vi "Create Summary File.vi"(7 "FP":T1, 8 "error in":errorcluster, 11 "Report":T2) -> (0 "error out":errorcluster, 1 "Vac?":bool, 2 "Pass/Fail":bool, 3 "resulting string":string)   [LabVIEW 2018]
uses:
  Results.ctl
  Vacuum Test.ctl
  Vacuum Output.ctl
  Main Refs.ctl
  Hardware/Tecan/Pump Config.ctl
  Vacuum Specs.ctl
  Cartridges.ctl
  Cartridge Status.ctl
  Commands.ctl
  Lib/Time/Wells.ctl
  Lib/Time/Bottles.ctl
  Process State.ctl
  Main Globals.vi
panel:
  # "Tecan Pump"
  # "Vacuum"
  # "General"
  # "Protocol"
  # "Zaber"
  # "NFC Reader 1"
  # "NFC  Reader 2"
  # "NFC Reader 3"
  # "NFC Reader 4"
  # "System"
  # "Cartridge Utitlies"
  # "Wells"
  # "times"
  # "from"
  # "State Machine"
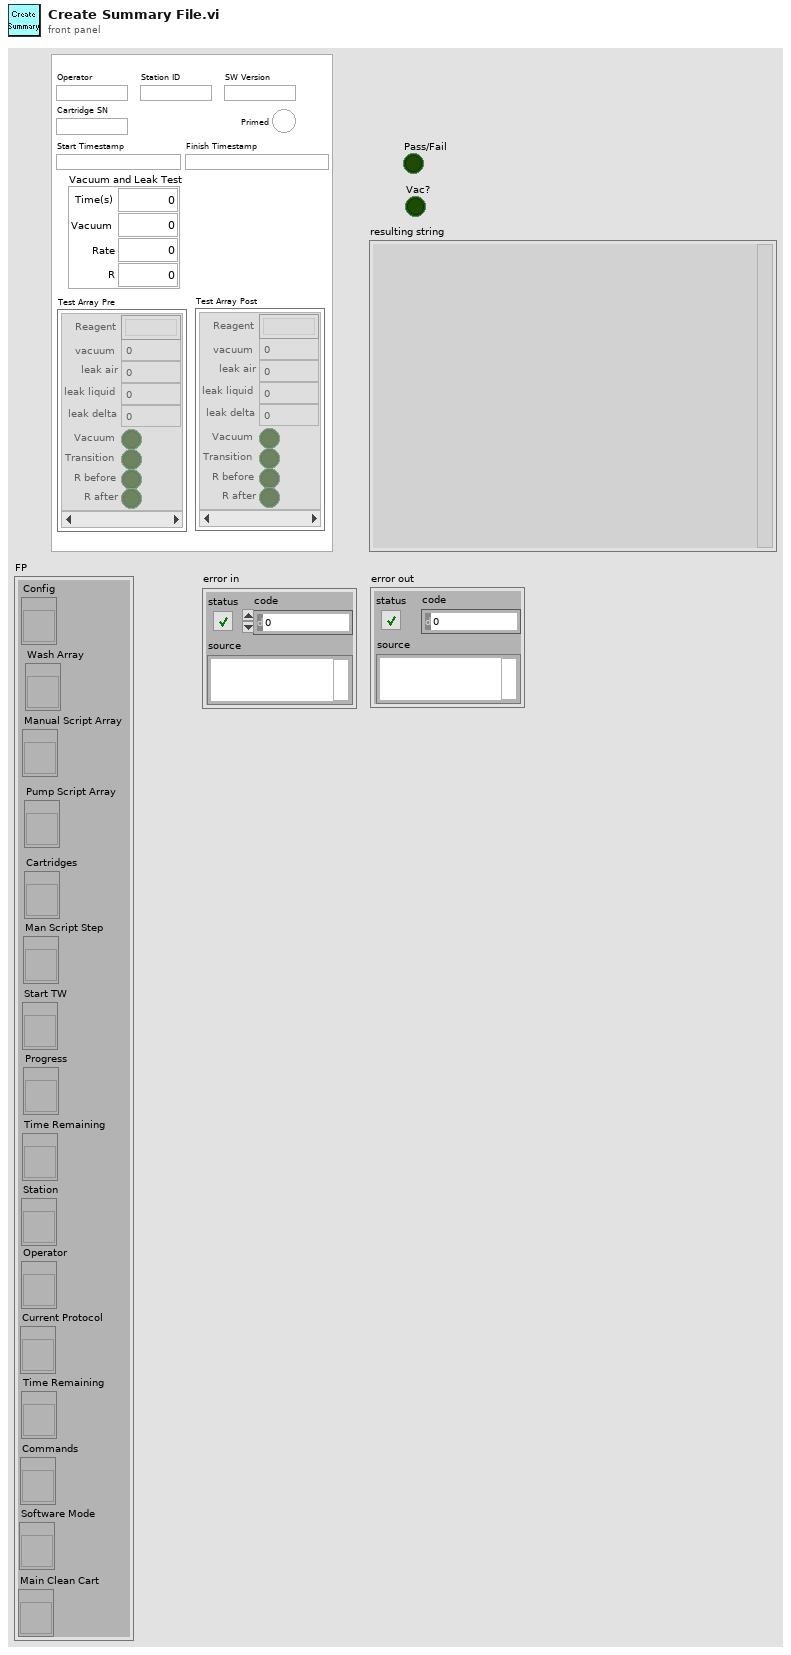
[diagram p1: front panel]
types:
  T1 = typedef "Main Refs.ctl" = cluster{"Config":refnum<vi>, "Wash Array":refnum<vi>, "Manual Script Array":refnum<vi>, "Pump Script Array":refnum<vi>, "Cartridges":refnum<vi>, "Man Script Step":refnum<vi>, "Start TW":refnum<vi>, "Progress":refnum<vi>, "Time Remaining":refnum<vi>, "Station":refnum<vi>, "Operator":refnum<vi>, "Current Protocol":refnum<vi>, "Time Remaining":refnum<vi>, "Commands":refnum<vi>, "Software Mode":refnum<vi>, "Main Clean Cart":refnum<vi>}
  T2 = typedef "Results.ctl" = cluster{"Operator":string, "Station ID":string, "SW Version":string, "Cartridge SN":string, "Primed":bool, "Start Timestamp":string, "Finish Timestamp":string, "Test Array Pre":T3[], "Test Array Post":T3[], "Vacuum and Leak Test":T4}
  T3 = typedef "Vacuum Test.ctl" = cluster{"vacuum":dbl, "leak air":dbl, "leak liquid":dbl, "leak delta":dbl, "Transition":bool, "Vacuum":bool, "R before":bool, "R after":bool, "Reagent":string}
  T4 = typedef "Vacuum Output.ctl" = cluster{"Time(s)":dbl, "Vacuum":dbl, "Rate":dbl, "R":dbl}
  T5 = enum16{"open", "replace", "create", "open or create", "replace or create", "replace or create with confirmation"}
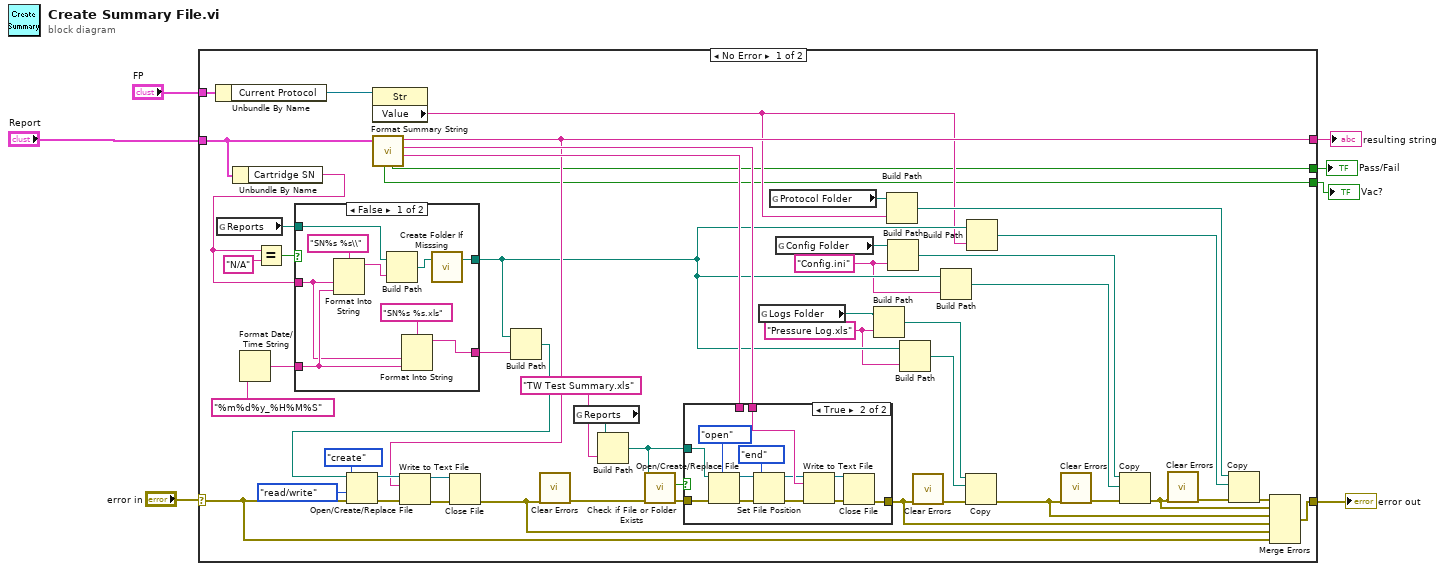
[diagram p0: block diagram]
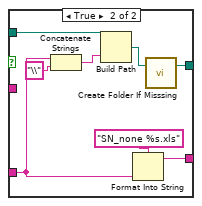
[diagram p2: hidden frame]
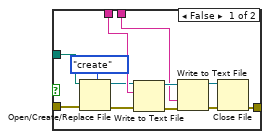
[diagram p3: hidden frame]
diagram:
  n1 = case shown="No Error" "error in" {
    selector: "error in" -> [w11 w100]
    tunnel: "Report" -> [w58 _]
    tunnel: [w15 w100] -> w6
    tunnel: [w45 _] -> w5
    tunnel: "FP" -> [w36 _]
    tunnel: [w9 _] -> w2
    tunnel: [w8 _] -> w1
    frame No Error {
      w28 = "Config.ini" ("name or relative path")
      w27 = "Pressure Log.xls" ("name or relative path")
      n2 = Unbundle By Name(w36) -> ("Current Protocol"=w35:refnum<vi>)
      n3 = global read "Main Globals.vi" "Reports"() -> (w24:path)
      n4 = Unbundle By Name(w58) -> ("Cartridge SN"=w23:string)
      n5 = Format Date/Time String(time format string (%c)="%m%d%y_%H%M%S") -> (date/time string=w25:string)  [unwired: 2 in]
      n6 = Equal?(x=w23, y="N/A") -> (x = y?=w21:bool)
      n7 = case shown="False" w21 {
        tunnel: [w66 w72] -> w32
        tunnel: w23 -> [w60 _]
        tunnel: w25 -> [w61 w68]
        tunnel: w24 -> [w65 w71]
        tunnel: [w59 w69] -> w20
        frame False {
          n8 = Format Into String(format string="SN%s %s\\", w60, w61) -> (resulting string=w63:string)  [unwired: 2 in, 1 out]
          n9 = Build Path(base path=w65, name or relative path=w63) -> (appended path=w67:path)
          n10 = Format Into String(format string="SN%s %s.xls", w60, w61) -> (resulting string=w59:string)  [unwired: 2 in, 1 out]
          n11 = call "Create Folder If Misssing.vi"("Path In"=w67) -> ("Path Out"=w66:path)  [unwired: 1 in, 1 out]
        }
        frame True {
          n12 = Concatenate Strings(w68, "\\" ("string")) -> (w74:string)
          n13 = Build Path(base path=w71, name or relative path=w74) -> (appended path=w73:path)
          n14 = Format Into String(format string="SN_none %s.xls", w68) -> (resulting string=w69:string)  [unwired: 2 in, 1 out]
          n15 = call "Create Folder If Misssing.vi"("Path In"=w73) -> ("Path Out"=w72:path)  [unwired: 1 in, 1 out]
        }
      }
      n16 = property class="Str"(reference=w35) -> ("Value"=w31:string)  [unwired: 1 in, 2 out]
      n17 = call "Format Summary String.vi"("Report"=w58) -> ("summary string header"=w50:string, "summary string"=w51:string, "full report string"=w45:string, "Transition?"=w9:bool, "Vac?"=w8:bool)  [unwired: 5 in, 1 out]
      n18 = Build Path(base path=w32, name or relative path=w20) -> (appended path=w48:path)
      n19 = Open/Create/Replace File(file path (use dialog)=w48, error in=w11, operation (0:open)=T5."create", access (0:read/write)=enum16{"read/write", "read-only", "write-only"}."read/write") -> (refnum out=w47:refnum<file>, error out=w46:errorcluster)  [unwired: 2 in, 1 out]
      n20 = Write to Text File(file (use dialog)=w47, text=w45, error in=w46) -> (refnum out=w43:refnum<file>, error out=w44:errorcluster)  [unwired: 1 in, 1 out]
      n21 = Close File(refnum=w43, error in=w44) -> (error out=w12:errorcluster)  [unwired: 1 out]
      n22 = call <vilib>:"Clear Errors.vi"("error in (no error)"=w12) -> ("error out"=w19:errorcluster)  [unwired: 5 in, 1 out]
      n23 = global read "Main Globals.vi" "Reports"() -> (w56:path)
      n24 = Build Path(base path=w56, name or relative path="TW Test Summary.xls") -> (appended path=w52:path)
      n25 = call <vilib>:"Check if File or Folder Exists.vi"("error in (no error)"=w19, "path"=w52) -> ("error out"=w54:errorcluster, "file or folder exists?"=w53:bool)  [unwired: 7 in, 1 out]
      n26 = case shown="True" w53 {
        tunnel: w54 -> [w86 w99]
        tunnel: w52 -> [w85 w98]
        tunnel: w51 -> [w79 w93]
        tunnel: [w77 w89] -> w13
        tunnel: w50 -> [w83 _]
        frame False {
          n27 = Open/Create/Replace File(file path (use dialog)=w85, error in=w86, operation (0:open)=T5."create") -> (refnum out=w82:refnum<file>, error out=w84:errorcluster)  [unwired: 3 in, 1 out]
          n28 = Write to Text File(file (use dialog)=w82, text=w83, error in=w84) -> (refnum out=w80:refnum<file>, error out=w81:errorcluster)  [unwired: 1 in, 1 out]
          n29 = Write to Text File(file (use dialog)=w80, text=w79, error in=w81) -> (refnum out=w76:refnum<file>, error out=w78:errorcluster)  [unwired: 1 in, 1 out]
          n30 = Close File(refnum=w76, error in=w78) -> (error out=w77:errorcluster)  [unwired: 1 out]
        }
        frame True {
          n31 = Open/Create/Replace File(file path (use dialog)=w98, error in=w99, operation (0:open)=T5."open") -> (refnum out=w96:refnum<file>, error out=w94:errorcluster)  [unwired: 3 in, 1 out]
          n32 = Set File Position(refnum=w96, from (0:start)=enum16{"start", "end", "current"}."end", error in=w94) -> (refnum out=w92:refnum<file>, error out=w91:errorcluster)  [unwired: 1 in]
          n33 = Write to Text File(file (use dialog)=w92, text=w93, error in=w91) -> (refnum out=w88:refnum<file>, error out=w90:errorcluster)  [unwired: 1 in, 1 out]
          n34 = Close File(refnum=w88, error in=w90) -> (error out=w89:errorcluster)  [unwired: 1 out]
        }
      }
      n35 = global read "Main Globals.vi" "Logs Folder"() -> (w41:path)
      n36 = global read "Main Globals.vi" "Protocol Folder"() -> (w34:path)
      n37 = global read "Main Globals.vi" "Config Folder"() -> (w39:path)
      n38 = Build Path(base path=w41, name or relative path=w27) -> (appended path=w26:path)
      n39 = Build Path(base path=w34, name or relative path=w31) -> (appended path=w33:path)
      n40 = Build Path(base path=w39, name or relative path=w28) -> (appended path=w38:path)
      n41 = Build Path(base path=w32, name or relative path=w27) -> (appended path=w40:path)
      n42 = call <vilib>:"Clear Errors.vi"("error in (no error)"=w13) -> ("error out"=w18:errorcluster)  [unwired: 5 in, 1 out]
      n43 = Build Path(base path=w32, name or relative path=w28) -> (appended path=w37:path)
      n44 = Copy(8:w18, 10:w40, 11:w26) -> (0:w10:errorcluster)  [unwired: 2 in, 2 out]
      n45 = Build Path(base path=w32, name or relative path=w31) -> (appended path=w30:path)
      n46 = call <vilib>:"Clear Errors.vi"("error in (no error)"=w10) -> ("error out"=w17:errorcluster)  [unwired: 5 in, 1 out]
      n47 = Copy(8:w17, 10:w37, 11:w38) -> (0:w14:errorcluster)  [unwired: 2 in, 2 out]
      n48 = call <vilib>:"Clear Errors.vi"("error in (no error)"=w14) -> ("error out"=w16:errorcluster)  [unwired: 5 in, 1 out]
      n49 = Copy(8:w16, 10:w30, 11:w33) -> (0:w29:errorcluster)  [unwired: 2 in, 2 out]
      n50 = Merge Errors(w29, w14, w10, w13, w12, w11) -> (w15:errorcluster)
    }
    frame Error {
    }
  }
  "error out" <- w6
  "resulting string" <- w5
  "Pass/Fail" <- w2
  "Vac?" <- w1
